vi "Find Values.vi"(9 "Response string":string, 10 "keys":string[](array[string])) -> (1 "values":string[](array[string]), 2 "keys dup":string[](array[string]))   [LabVIEW 2013, in "Oauth2.lvclass"]
uses:
  Oauth2.lvclass
  <vilib>/LabVIEW Open Source Project/OpenURI/openURI.lvlib
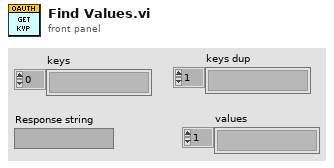
[diagram p1: front panel]
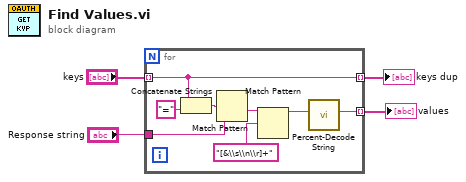
[diagram p0: block diagram]
diagram:
  n1 = for {
    tunnel: "Response string" -> [w12]
    tunnel: [w5] -> w3 mode=indexing
    tunnel: "keys" -> [w7] mode=indexing
    tunnel: [w7] -> w1 mode=indexing
    n2 = Concatenate Strings(w7, "=" ("regular expression")) -> (w8:string)
    n3 = Match Pattern(string=w12, regular expression=w8) -> (after substring=w11:string)  [unwired: 1 in, 3 out]
    n4 = Match Pattern(string=w11, regular expression="[&\\s\\n\\r]+") -> (before substring=w6:string)  [unwired: 1 in, 3 out]
    n5 = call <vilib>:"Percent-Decode String.vi"("Pct-Encoded String"=w6) -> ("String"=w5:string)  [unwired: 10 in]
  }
  "values" <- w3
  "keys dup" <- w1
